vi "Get Address Map Element.vi"(2 "Basecard Config Registers":refnum<class "7902R Basecard Config Registers.lvclass">, 5 "index":u8) -> (6 "address map element":T1)   [LabVIEW 2019, in "7902R Basecard Config Registers.lvclass"]
uses:
  7902R Basecard Config Registers.lvclass
  <instrlib>/_niInstr/Instruction Framework/v1/FPGA/Typedefs/Address Map Element.ctl
  <instrlib>/_niInstr/Instruction Framework/v1/FPGA/Typedefs/niInstr Instruction Framework v1 FPGA.lvlib
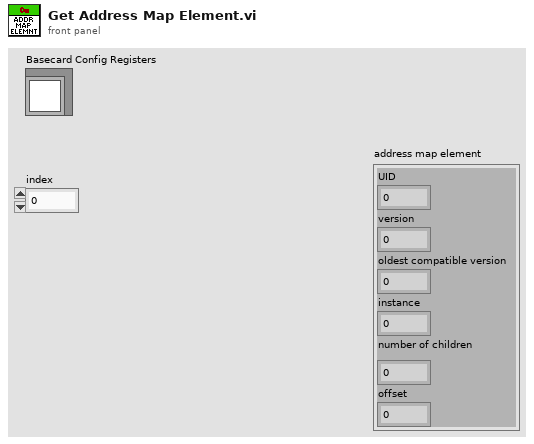
[diagram p1: front panel]
types:
  T1 = typedef "niInstr Instruction Framework v1 FPGA.lvlib/Address Map Element.ctl" = cluster{"UID":u16, "version":u16, "oldest compatible version":u16, "instance":u8, "number of children":u8, "offset":u32}
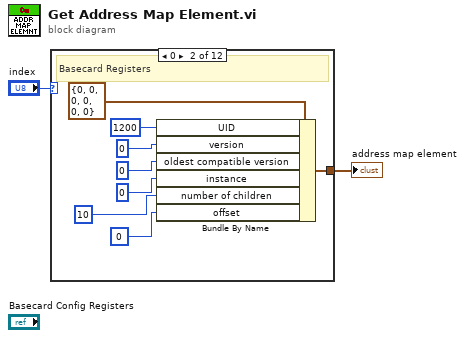
[diagram p0: block diagram]
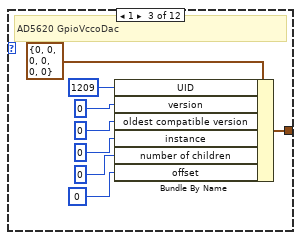
[diagram p3: hidden frame]
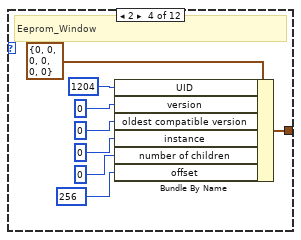
[diagram p4: hidden frame]
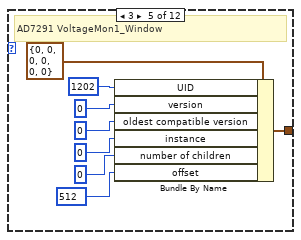
[diagram p5: hidden frame]
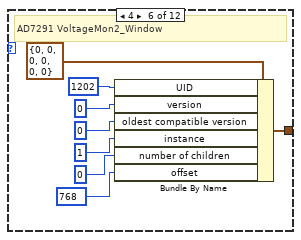
[diagram p6: hidden frame]
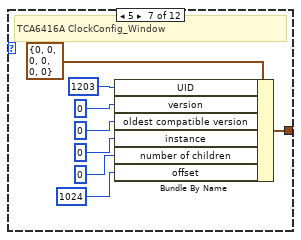
[diagram p7: hidden frame]
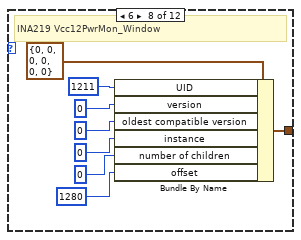
[diagram p8: hidden frame]
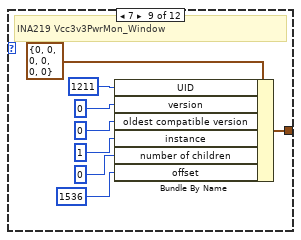
[diagram p9: hidden frame]
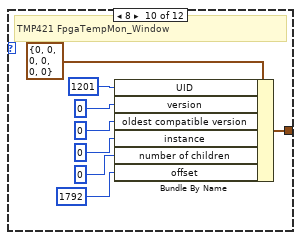
[diagram p10: hidden frame]
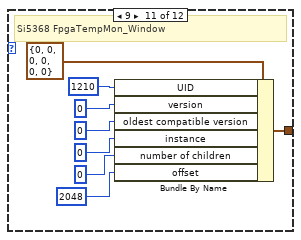
[diagram p11: hidden frame]
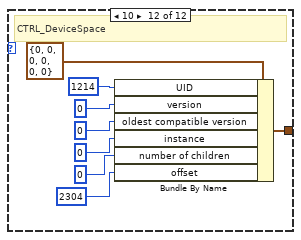
[diagram p12: hidden frame]
diagram:
  n1 = case shown="0" "index" {
    tunnel: [_ w9 w17 w25 w33 w41 w49 w57 w65 w73 w81 w89] -> w1
    frame Default {
    }
    frame 0 {
      # "Basecard Registers"
      n2 = Bundle By Name(cluster=T1 {"UID"=0, "version"=0, "oldest compatible version"=0, "instance"=0, "number of children"=0, "offset"=0} ("address map element"), "UID"=u16 1200, "version"=u16 0, "oldest compatible version"=u16 0, "instance"=u8 0, "number of children"=u8 10, "offset"=u32 0) -> (w9:T1)
    }
    frame 1 {
      # "AD5620 GpioVccoDac"
      n3 = Bundle By Name(cluster=T1 {"UID"=0, "version"=0, "oldest compatible version"=0, "instance"=0, "number of children"=0, "offset"=0} ("address map element"), "UID"=u16 1209, "version"=u16 0, "oldest compatible version"=u16 0, "instance"=u8 0, "number of children"=u8 0, "offset"=u32 0) -> (w17:T1)
    }
    frame 2 {
      # "Eeprom_Window"
      n4 = Bundle By Name(cluster=T1 {"UID"=0, "version"=0, "oldest compatible version"=0, "instance"=0, "number of children"=0, "offset"=0} ("address map element"), "UID"=u16 1204, "version"=u16 0, "oldest compatible version"=u16 0, "instance"=u8 0, "number of children"=u8 0, "offset"=u32 256) -> (w25:T1)
    }
    frame 3 {
      # "AD7291 VoltageMon1_Window"
      n5 = Bundle By Name(cluster=T1 {"UID"=0, "version"=0, "oldest compatible version"=0, "instance"=0, "number of children"=0, "offset"=0} ("address map element"), "UID"=u16 1202, "version"=u16 0, "oldest compatible version"=u16 0, "instance"=u8 0, "number of children"=u8 0, "offset"=u32 512) -> (w33:T1)
    }
    frame 4 {
      # "AD7291 VoltageMon2_Window"
      n6 = Bundle By Name(cluster=T1 {"UID"=0, "version"=0, "oldest compatible version"=0, "instance"=0, "number of children"=0, "offset"=0} ("address map element"), "UID"=u16 1202, "version"=u16 0, "oldest compatible version"=u16 0, "instance"=u8 1, "number of children"=u8 0, "offset"=u32 768) -> (w41:T1)
    }
    frame 5 {
      # "TCA6416A ClockConfig_Window"
      n7 = Bundle By Name(cluster=T1 {"UID"=0, "version"=0, "oldest compatible version"=0, "instance"=0, "number of children"=0, "offset"=0} ("address map element"), "UID"=u16 1203, "version"=u16 0, "oldest compatible version"=u16 0, "instance"=u8 0, "number of children"=u8 0, "offset"=u32 1024) -> (w49:T1)
    }
    frame 6 {
      # "INA219 Vcc12PwrMon_Window"
      n8 = Bundle By Name(cluster=T1 {"UID"=0, "version"=0, "oldest compatible version"=0, "instance"=0, "number of children"=0, "offset"=0} ("address map element"), "UID"=u16 1211, "version"=u16 0, "oldest compatible version"=u16 0, "instance"=u8 0, "number of children"=u8 0, "offset"=u32 1280) -> (w57:T1)
    }
    frame 7 {
      # "INA219 Vcc3v3PwrMon_Window"
      n9 = Bundle By Name(cluster=T1 {"UID"=0, "version"=0, "oldest compatible version"=0, "instance"=0, "number of children"=0, "offset"=0} ("address map element"), "UID"=u16 1211, "version"=u16 0, "oldest compatible version"=u16 0, "instance"=u8 1, "number of children"=u8 0, "offset"=u32 1536) -> (w65:T1)
    }
    frame 8 {
      # "TMP421 FpgaTempMon_Window"
      n10 = Bundle By Name(cluster=T1 {"UID"=0, "version"=0, "oldest compatible version"=0, "instance"=0, "number of children"=0, "offset"=0} ("address map element"), "UID"=u16 1201, "version"=u16 0, "oldest compatible version"=u16 0, "instance"=u8 0, "number of children"=u8 0, "offset"=u32 1792) -> (w73:T1)
    }
    frame 9 {
      # "Si5368 FpgaTempMon_Window"
      n11 = Bundle By Name(cluster=T1 {"UID"=0, "version"=0, "oldest compatible version"=0, "instance"=0, "number of children"=0, "offset"=0} ("address map element"), "UID"=u16 1210, "version"=u16 0, "oldest compatible version"=u16 0, "instance"=u8 0, "number of children"=u8 0, "offset"=u32 2048) -> (w81:T1)
    }
    frame 10 {
      # "CTRL_DeviceSpace"
      n12 = Bundle By Name(cluster=T1 {"UID"=0, "version"=0, "oldest compatible version"=0, "instance"=0, "number of children"=0, "offset"=0} ("address map element"), "UID"=u16 1214, "version"=u16 0, "oldest compatible version"=u16 0, "instance"=u8 0, "number of children"=u8 0, "offset"=u32 2304) -> (w89:T1)
    }
  }
  "address map element" <- w1
